vi "DAC Configure.vi"(8 "error in":errorcluster, 11 "DAC Traverse in":refnum<class "DAC Traverse.lvclass">) -> (0 "error out":errorcluster, 3 "DAC Traverse out":refnum<class "DAC Traverse.lvclass">)   [LabVIEW 2019, in "DAC.lvlib" / "DAC Traverse.lvclass"]
uses:
  DAC Traverse.lvclass
  DAC.lvclass
  <vilib>/Instr/_visa.llb/VISA Configure Serial Port (Instr).vi
  C:/Users/wg/Documents/LV_Projects/test-stand/App/DAC/DAC.lvclass
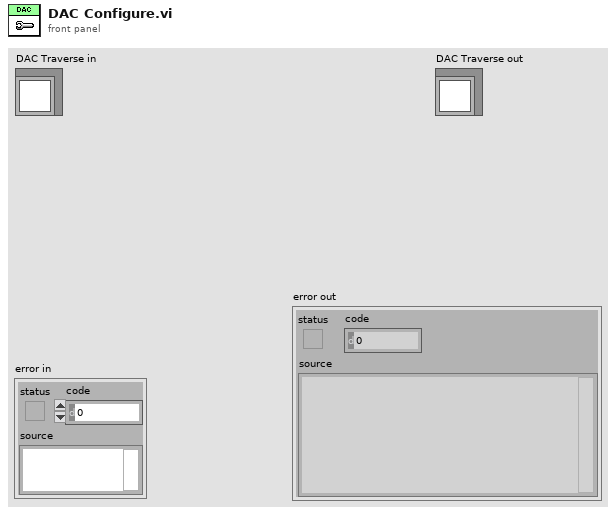
[diagram p1: front panel]
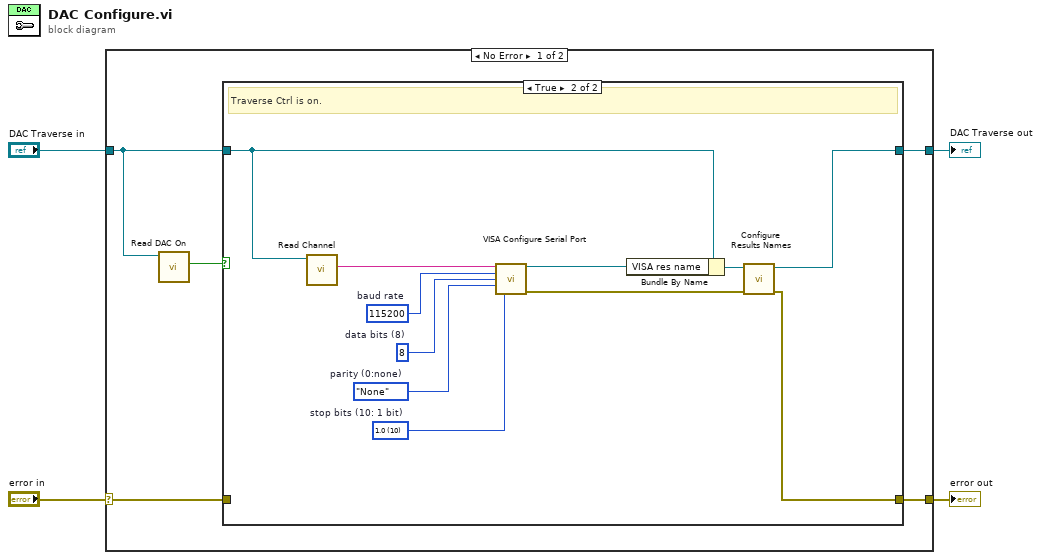
[diagram p0: block diagram]
diagram:
  n1 = case shown="No Error" "error in" {
    selector: "error in" -> [w6 w24]
    tunnel: [w5 w24] -> w4
    tunnel: [w7 w23] -> w3
    tunnel: "DAC Traverse in" -> [w9 w23]
    frame No Error {
      n2 = call "Read DAC On.vi"("DAC in"=w9) -> ("DAC On"=w8:bool)  [unwired: 8 in, 2 out]
      n3 = case shown="True" w8 {
        tunnel: w9 -> [w11 w13]
        tunnel: [w11 w22] -> w7
        tunnel: w6 -> [w10 _]
        tunnel: [w10 w19] -> w5
        frame False {
          # "Traverse Ctrl is off."
        }
        frame True {
          w15 = u16 10 items=["1.0"=10, "1.5"=15, "2.0"=20]  # stop bits (10: 1 bit)
          w16 = enum16{"None", "Odd", "Even", "Mark", "Space"}."None"  # parity (0:none)
          w17 = u16 8  # data bits (8)
          w18 = u32 115200  # baud rate
          # "Traverse Ctrl is on."
          n4 = call "Read Channel.vi"("DAC in"=w13) -> ("Channel"=w12:string)  [unwired: 8 in, 2 out]
          n5 = call-poly "VISA Configure Serial Port"("VISA resource name"=w12, "baud rate (9600)"=w18, "data bits (8)"=w17, "parity (0:none)"=w16, "stop bits (10: 1 bit)"=w15) -> ("VISA resource name out"=w14:refnum<visa-resource-name>, "error out"=w20:errorcluster)  [unwired: 9 in]
          n6 = Bundle By Name(cluster=w13, "VISA res name"=w14) -> (w21:refnum<class "DAC Traverse.lvclass">)
          n7 = call "Configure Results Names.vi"("error in"=w20, "DAC Traverse in"=w21) -> ("error out"=w19:errorcluster, "DAC Traverse out"=w22:refnum<class "DAC Traverse.lvclass">)  [unwired: 8 in]
        }
      }
    }
    frame Error {
    }
  }
  "error out" <- w4
  "DAC Traverse out" <- w3
